vi "Linear Resistance.vi"(1 "Current":dbl[](array[numeric]), 2 "Voltage":dbl[](array[numeric])) -> (0 "Resistance":dbl)   [LabVIEW 2013]
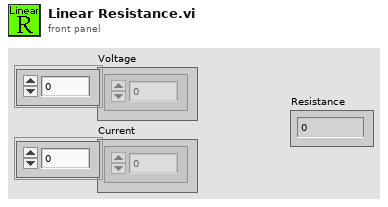
[diagram p1: front panel]
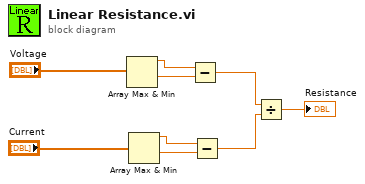
[diagram p0: block diagram]
diagram:
  n1 = Array Max & Min(array="Voltage") -> (max value=w8:dbl, min value=w7:dbl)  [unwired: 2 out]
  n2 = Array Max & Min(array="Current") -> (max value=w6:dbl, min value=w5:dbl)  [unwired: 2 out]
  n3 = Subtract(x=w8, y=w7) -> (x-y=w3:dbl)
  n4 = Subtract(x=w6, y=w5) -> (x-y=w2:dbl)
  n5 = Divide(x=w3, y=w2) -> (x/y=→"Resistance":dbl)
